vi "PH_BackreflectionMeas.create waveform.vi"(1 "dt":dbl, 2 "Y-Data":dbl[](array[numeric])) -> (0 "waveform out":waveform(dbl))   [LabVIEW 2014, in "PH_BackreflectionMeas.lvlib"]
uses:
  PH_BackreflectionMeas.lvlib
  <vilib>/Waveform/WDTOps.llb/WDT Get Waveform Subset DBL.vi
  <vilib>/measure/madcrms.llb/Basic Averaged DC-RMS for 1 Chan.vi
  <vilib>/measure/NI_MAPro.lvlib
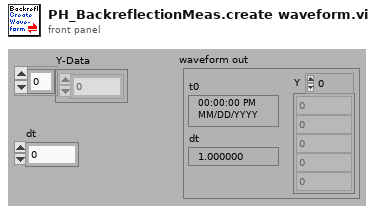
[diagram p1: front panel]
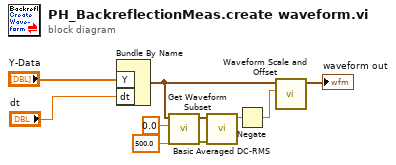
[diagram p0: block diagram]
diagram:
  n1 = Bundle By Name("Y"="Y-Data", "dt"="dt") -> (w1:waveform(dbl))  [unwired: 1 in]
  n2 = call-poly <vilib>:"Get Waveform Subset.vi"("duration"=500.0, "start samples/time"=0.0, "waveform in"=w1) -> ("error out"=w2:errorcluster, "waveform out"=w3:waveform(dbl))  [unwired: 3 in, 2 out]
  n3 = call-poly <vilib>:"Basic Averaged DC-RMS.vi"("error in (no error)"=w2, "signal in"=w3) -> ("DC value"=w6:dbl)  [unwired: 6 in, 3 out]
  n4 = Negate(x=w6) -> (-x=w7:dbl)
  n5 = call <vilib>:"Waveform Scale and Offset.vi"("offset"=w7, "waveform in"=w1) -> ("waveform out"=→"waveform out":waveform(dbl))  [unwired: 8 in, 1 out]
